vi "3D Primitive Data.vi"(10 "Normal Binding Mode":T1(ring), 11 "Primitive Mode":T3(ring)) -> (1 "Normal Array":cluster{"X":sgl, "Y":sgl, "Z":sgl}[](array[cluster]), 2 "Indices":u32[](array[numeric]), 3 "Vertex Array":cluster{"X":sgl, "Y":sgl, "Z":sgl}[](array[cluster]), 4 "Texture Array":cluster{"X":sgl, "Y":sgl}[](array[cluster]), 5 "Color Array":T2(array[cluster]))   [LabVIEW 2023]
doc: "Create meshes of points for the Using Meshes.vi example. Define some known parameters so the mesh can be processed."
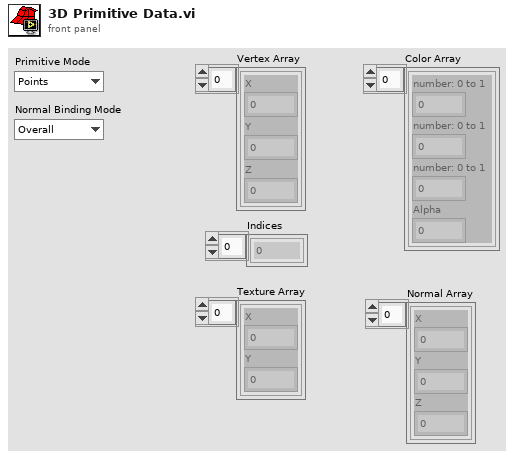
[diagram p1: front panel]
types:
  T1 = enum16{"Overall", "Per Primitive", "Per Vertex", "Binding Off"}
  T2 = cluster{"number: 0 to 1":dbl, "number: 0 to 1":dbl, "number: 0 to 1":dbl, "Alpha":dbl}[]
  T3 = enum16{"Points", "Lines", "Line Strip", "Line Loop", "Triangles", "Triangle Strip", "Triangle Fan", "Quads", "Quad Strip", "Polygon"}
  T4 = cluster{"number: 0 to 1":dbl, "number: 0 to 1":dbl, "number: 0 to 1":dbl}
  T5 = cluster{"number: 0 to 1":dbl, "number: 0 to 1":dbl, "number: 0 to 1":dbl, dbl}
  T6 = cluster{"number: 0 to 1":dbl, "number: 0 to 1":dbl, "number: 0 to 1":dbl, dbl}[]
  T7 = cluster{"number: 0 to 1":dbl, "number: 0 to 1":dbl, "number: 0 to 1":dbl}[]
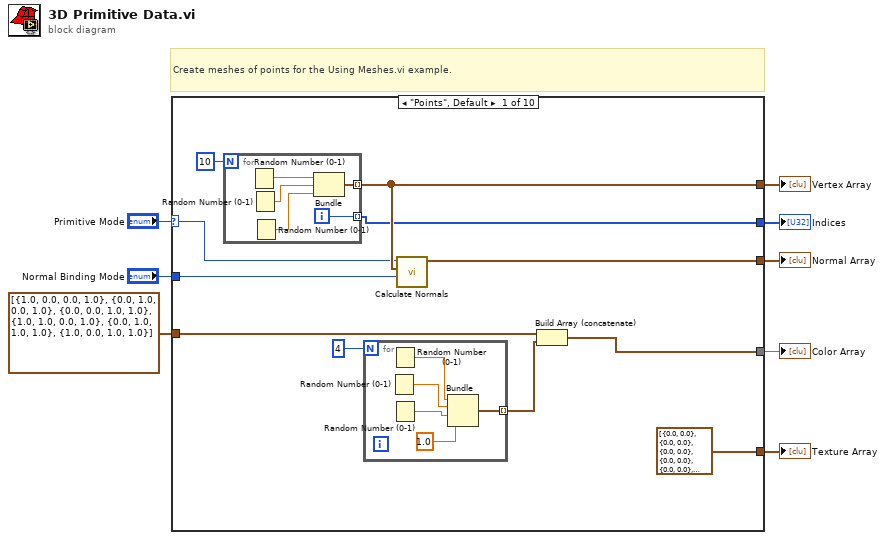
[diagram p0: block diagram]
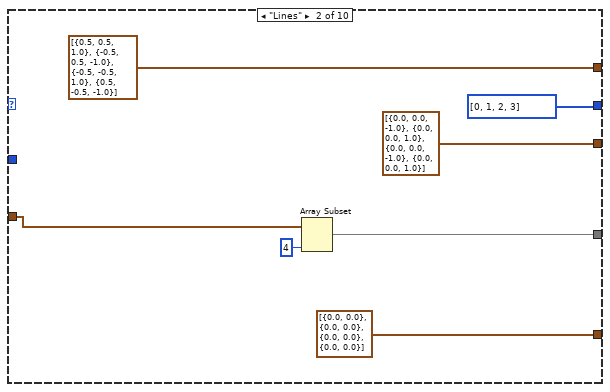
[diagram p2: hidden frame]
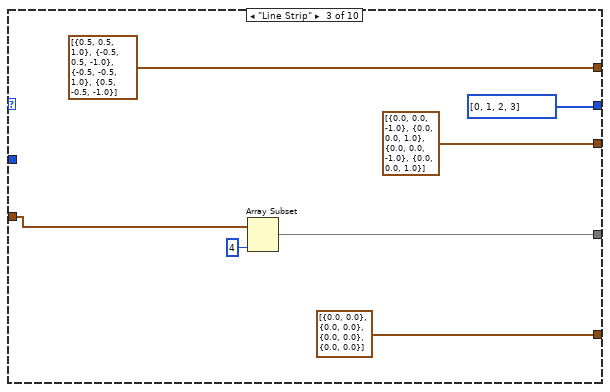
[diagram p3: hidden frame]
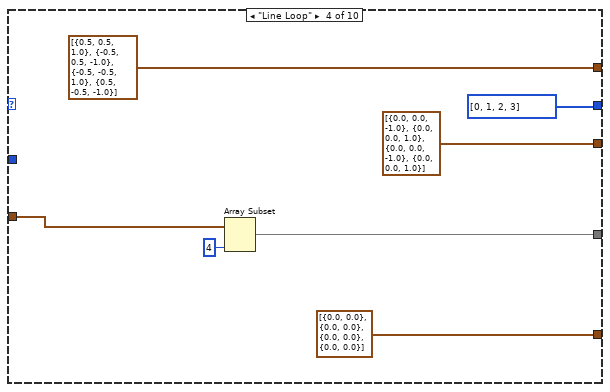
[diagram p4: hidden frame]
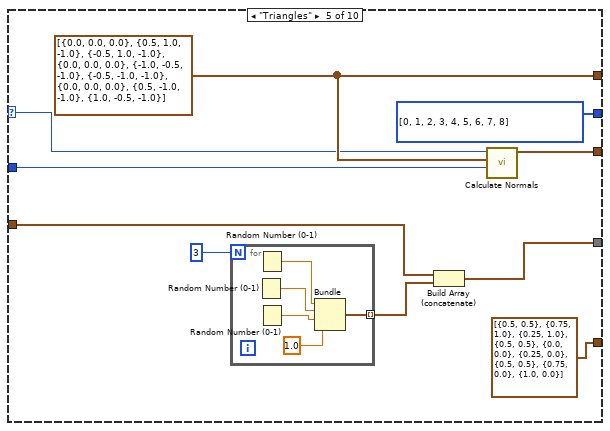
[diagram p5: hidden frame]
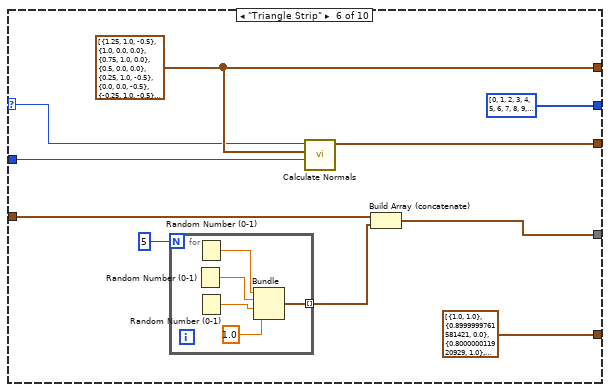
[diagram p6: hidden frame]
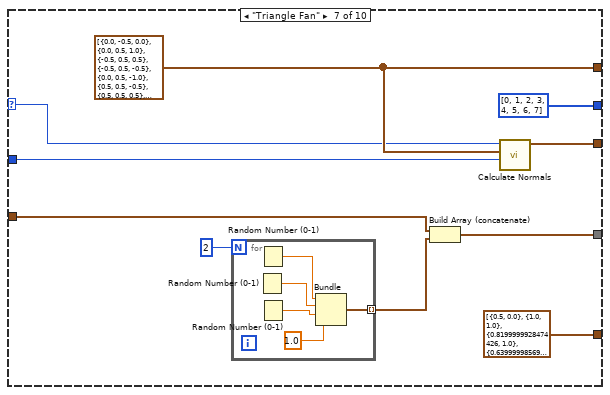
[diagram p7: hidden frame]
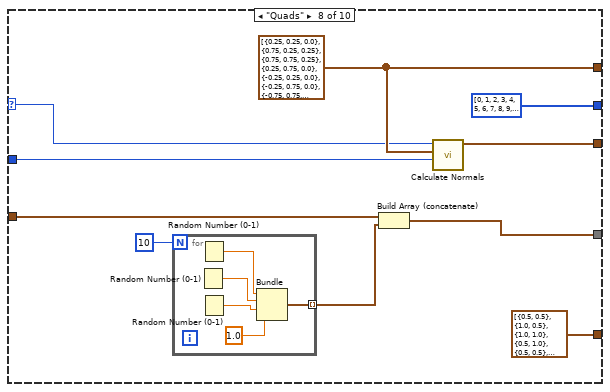
[diagram p8: hidden frame]
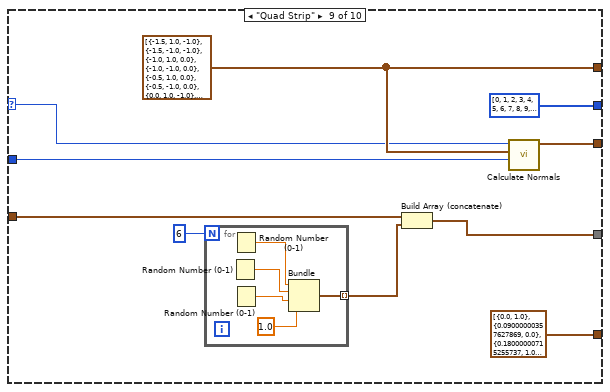
[diagram p9: hidden frame]
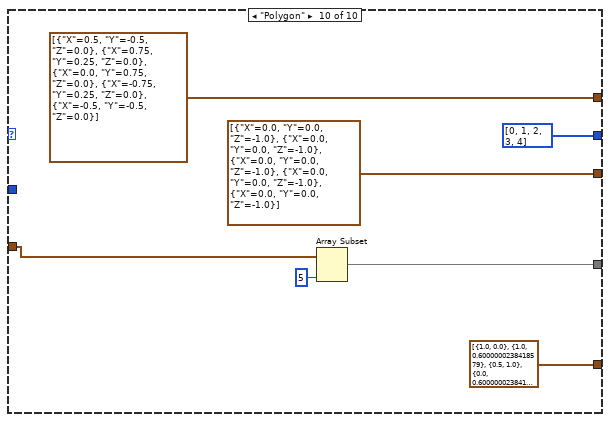
[diagram p10: hidden frame]
diagram:
  # "Create meshes of points for the Using Meshes.vi example."
  n1 = case shown="\"Points\", Default" "Primitive Mode" {
    selector: "Primitive Mode" -> [w9 _ _ _ w51 w66 w81 w96 w111 _]
    tunnel: [w19 cluster{"X":sgl, "Y":sgl, "Z":sgl}[] [{"X"=0.0, "Y"=0.0, "Z"=-1.0}, {"X"=0.0, "Y"=0.0, "Z"=1.0}, {"X"=0.0, "Y"=0.0, "Z"=-1.0}, {"X"=0.0, "Y"=0.0, "Z"=1.0}] cluster{"X":sgl, "Y":sgl, "Z":sgl}[] [{"X"=0.0, "Y"=0.0, "Z"=-1.0}, {"X"=0.0, "Y"=0.0, "Z"=1.0}, {"X"=0.0, "Y"=0.0, "Z"=-1.0}, {"X"=0.0, "Y"=0.0, "Z"=1.0}] cluster{"X":sgl, "Y":sgl, "Z":sgl}[] [{"X"=0.0, "Y"=0.0, "Z"=-1.0}, {"X"=0.0, "Y"=0.0, "Z"=1.0}, {"X"=0.0, "Y"=0.0, "Z"=-1.0}, {"X"=0.0, "Y"=0.0, "Z"=1.0}] w58 w73 w88 w103 w117 cluster{"X":sgl, "Y":sgl, "Z":sgl}[] [{"X"=0.0, "Y"=0.0, "Z"=-1.0}, {"X"=0.0, "Y"=0.0, "Z"=-1.0}, {"X"=0.0, "Y"=0.0, "Z"=-1.0}, {"X"=0.0, "Y"=0.0, "Z"=-1.0}, {"X"=0.0, "Y"=0.0, "Z"=-1.0}]] -> w8
    tunnel: [w17 cluster{"X":sgl, "Y":sgl, "Z":sgl}[] [{"X"=0.5, "Y"=0.5, "Z"=1.0}, {"X"=-0.5, "Y"=0.5, "Z"=-1.0}, {"X"=-0.5, "Y"=-0.5, "Z"=1.0}, {"X"=0.5, "Y"=-0.5, "Z"=-1.0}] ("Vertex Array") cluster{"X":sgl, "Y":sgl, "Z":sgl}[] [{"X"=0.5, "Y"=0.5, "Z"=1.0}, {"X"=-0.5, "Y"=0.5, "Z"=-1.0}, {"X"=-0.5, "Y"=-0.5, "Z"=1.0}, {"X"=0.5, "Y"=-0.5, "Z"=-1.0}] ("Vertex Array") cluster{"X":sgl, "Y":sgl, "Z":sgl}[] [{"X"=0.5, "Y"=0.5, "Z"=1.0}, {"X"=-0.5, "Y"=0.5, "Z"=-1.0}, {"X"=-0.5, "Y"=-0.5, "Z"=1.0}, {"X"=0.5, "Y"=-0.5, "Z"=-1.0}] ("Vertex Array") w57 w74 w87 w102 w118 cluster{"X":sgl, "Y":sgl, "Z":sgl}[] [{"X"=0.5, "Y"=-0.5, "Z"=0.0}, {"X"=0.75, "Y"=0.25, "Z"=0.0}, {"X"=0.0, "Y"=0.75, "Z"=0.0}, {"X"=-0.75, "Y"=0.25, "Z"=0.0}, {"X"=-0.5, "Y"=-0.5, "Z"=0.0}] ("Vertex Array")] -> w6
    tunnel: [w10 w30 w37 w44 w54 w67 w83 w97 w112 w126] -> w5
    tunnel: [cluster{"X":sgl, "Y":sgl}[] [{"X"=0.0, "Y"=0.0}, {"X"=0.0, "Y"=0.0}, {"X"=0.0, "Y"=0.0}, {"X"=0.0, "Y"=0.0}, {"X"=0.0, "Y"=0.0}, {"X"=0.0, "Y"=0.0}, {"X"=0.0, "Y"=0.0}, {"X"=0.0, "Y"=0.0}, {"X"=0.0, "Y"=0.0}, {"X"=0.0, "Y"=0.0}] ("Texture Array") cluster{"X":sgl, "Y":sgl}[] [{"X"=0.0, "Y"=0.0}, {"X"=0.0, "Y"=0.0}, {"X"=0.0, "Y"=0.0}, {"X"=0.0, "Y"=0.0}] ("Vertex Array") cluster{"X":sgl, "Y":sgl}[] [{"X"=0.0, "Y"=0.0}, {"X"=0.0, "Y"=0.0}, {"X"=0.0, "Y"=0.0}, {"X"=0.0, "Y"=0.0}] ("Vertex Array") cluster{"X":sgl, "Y":sgl}[] [{"X"=0.0, "Y"=0.0}, {"X"=0.0, "Y"=0.0}, {"X"=0.0, "Y"=0.0}, {"X"=0.0, "Y"=0.0}] ("Vertex Array") cluster{"X":sgl, "Y":sgl}[] [{"X"=0.5, "Y"=0.5}, {"X"=0.75, "Y"=1.0}, {"X"=0.25, "Y"=1.0}, {"X"=0.5, "Y"=0.5}, {"X"=0.0, "Y"=0.0}, {"X"=0.25, "Y"=0.0}, {"X"=0.5, "Y"=0.5}, {"X"=0.75, "Y"=0.0}, {"X"=1.0, "Y"=0.0}] ("Vertex Array") cluster{"X":sgl, "Y":sgl}[] [{"X"=1.0, "Y"=1.0}, {"X"=0.9, "Y"=0.0}, {"X"=0.8, "Y"=1.0}, {"X"=0.7, "Y"=0.0}, {"X"=0.6, "Y"=1.0}, {"X"=0.5, "Y"=0.0}, {"X"=0.4, "Y"=1.0}, {"X"=0.3, "Y"=0.0}, {"X"=0.2, "Y"=1.0}, {"X"=0.1, "Y"=0.0}, {"X"=0.0, "Y"=1.0}] ("Vertex Array") cluster{"X":sgl, "Y":sgl}[] [{"X"=0.5, "Y"=0.0}, {"X"=1.0, "Y"=1.0}, {"X"=0.82, "Y"=1.0}, {"X"=0.64, "Y"=1.0}, {"X"=0.48, "Y"=1.0}, {"X"=0.32, "Y"=1.0}, {"X"=0.16, "Y"=1.0}, {"X"=1.0, "Y"=1.0}] ("Vertex Array") cluster{"X":sgl, "Y":sgl}[] [{"X"=0.5, "Y"=0.5}, {"X"=1.0, "Y"=0.5}, {"X"=1.0, "Y"=1.0}, {"X"=0.5, "Y"=1.0}, {"X"=0.5, "Y"=0.5}, {"X"=0.5, "Y"=1.0}, {"X"=0.0, "Y"=1.0}, {"X"=0.0, "Y"=0.5}, {"X"=0.5, "Y"=0.5}, {"X"=0.0, "Y"=0.5}, {"X"=0.0, "Y"=0.0}, {"X"=0.5, "Y"=0.0}, {"X"=0.5, "Y"=0.5}, {"X"=0.5, "Y"=0.0}, {"X"=1.0, "Y"=0.0}, {"X"=1.0, "Y"=0.5}] ("Vertex Array") cluster{"X":sgl, "Y":sgl}[] [{"X"=0.0, "Y"=1.0}, {"X"=0.09, "Y"=0.0}, {"X"=0.18, "Y"=1.0}, {"X"=0.27, "Y"=0.0}, {"X"=0.36, "Y"=1.0}, {"X"=0.45, "Y"=0.0}, {"X"=0.54, "Y"=1.0}, {"X"=0.63, "Y"=0.0}, {"X"=0.72, "Y"=1.0}, {"X"=0.81, "Y"=0.0}, {"X"=0.9, "Y"=1.0}, {"X"=1.0, "Y"=0.0}] ("Vertex Array") cluster{"X":sgl, "Y":sgl}[] [{"X"=1.0, "Y"=0.0}, {"X"=1.0, "Y"=0.6}, {"X"=0.5, "Y"=1.0}, {"X"=0.0, "Y"=0.6}, {"X"=0.0, "Y"=0.0}] ("Vertex Array")] -> w4
    tunnel: [w15 u32[] [0, 1, 2, 3] ("Indices") u32[] [0, 1, 2, 3] ("Indices") u32[] [0, 1, 2, 3] ("Indices") u32[] [0, 1, 2, 3, 4, 5, 6, 7, 8] ("Indices") u32[] [0, 1, 2, 3, 4, 5, 6, 7, 8, 9, 10] ("Indices") u32[] [0, 1, 2, 3, 4, 5, 6, 7] ("Indices") u32[] [0, 1, 2, 3, 4, 5, 6, 7, 8, 9, 10, 11, 12, 13, 14, 15] ("Indices") u32[] [0, 1, 2, 3, 4, 5, 6, 7, 8, 9, 10, 11] ("Indices") u32[] [0, 1, 2, 3, 4] ("Indices")] -> w3
    tunnel: "Normal Binding Mode" -> [w14 _ _ _ w55 w71 w86 w101 w116 _]
    tunnel: cluster{dbl, dbl, dbl, dbl}[] [{1.0, 0.0, 0.0, 1.0}, {0.0, 1.0, 0.0, 1.0}, {0.0, 0.0, 1.0, 1.0}, {1.0, 1.0, 0.0, 1.0}, {0.0, 1.0, 1.0, 1.0}, {1.0, 0.0, 1.0, 1.0}] -> [w13 w32 w39 w46 w53 w69 w84 w99 w114 w128]
    frame "Points", Default {
      n2 = for {
        N: 10 -> [_]
        tunnel: [w27] -> w17 mode=indexing
        tunnel: [w26] -> w15 mode=indexing
        i -> [w26]
        n3 = Random Number (0-1)() -> (number: 0 to 1=w29:dbl)
        n4 = Random Number (0-1)() -> (number: 0 to 1=w28:dbl)
        n5 = Random Number (0-1)() -> (number: 0 to 1=w25:dbl)
        n6 = Bundle("number: 0 to 1"=w29, "number: 0 to 1"=w28, "number: 0 to 1"=w25) -> (w27:T4)  [unwired: 1 in]
      }
      n7 = for {
        N: 4 -> [_]
        tunnel: [w24] -> w11 mode=indexing
        n8 = Random Number (0-1)() -> (number: 0 to 1=w21:dbl)
        n9 = Random Number (0-1)() -> (number: 0 to 1=w22:dbl)
        n10 = Random Number (0-1)() -> (number: 0 to 1=w20:dbl)
        n11 = Bundle("number: 0 to 1"=w22, "number: 0 to 1"=w21, "number: 0 to 1"=w20, 1.0) -> (w24:T5)  [unwired: 1 in]
      }
      n12 = call "Calculate Normals.vi"("Color Binding Mode"=w14, "Vertex Array"=w17, "Draw Mode"=w9) -> ("Normal Array"=w19:cluster{"X":sgl, "Y":sgl, "Z":sgl}[])  [unwired: 8 in]
      n13 = Build Array (concatenate)(w13, w11) -> (w10:T6)
    }
    frame "Lines" {
      n14 = Array Subset(array=w32, length=4) -> (w30:cluster{dbl, dbl, dbl, dbl}[])  [unwired: 1 in]
    }
    frame "Line Strip" {
      n15 = Array Subset(array=w39, length=4) -> (w37:cluster{dbl, dbl, dbl, dbl}[])  [unwired: 1 in]
    }
    frame "Line Loop" {
      n16 = Array Subset(array=w46, length=4) -> (w44:cluster{dbl, dbl, dbl, dbl}[])  [unwired: 1 in]
    }
    frame "Triangles" {
      w57 = cluster{"X":sgl, "Y":sgl, "Z":sgl}[] [{"X"=0.0, "Y"=0.0, "Z"=0.0}, {"X"=0.5, "Y"=1.0, "Z"=-1.0}, {"X"=-0.5, "Y"=1.0, "Z"=-1.0}, {"X"=0.0, "Y"=0.0, "Z"=0.0}, {"X"=-1.0, "Y"=-0.5, "Z"=-1.0}, {"X"=-0.5, "Y"=-1.0, "Z"=-1.0}, {"X"=0.0, "Y"=0.0, "Z"=0.0}, {"X"=0.5, "Y"=-1.0, "Z"=-1.0}, {"X"=1.0, "Y"=-0.5, "Z"=-1.0}] ("Vertex Array")
      n17 = for {
        N: 3 -> [_]
        tunnel: [w65] -> w52 mode=indexing
        n18 = Random Number (0-1)() -> (number: 0 to 1=w62:dbl)
        n19 = Random Number (0-1)() -> (number: 0 to 1=w63:dbl)
        n20 = Random Number (0-1)() -> (number: 0 to 1=w61:dbl)
        n21 = Bundle("number: 0 to 1"=w63, "number: 0 to 1"=w62, "number: 0 to 1"=w61, 1.0) -> (w65:T5)  [unwired: 1 in]
      }
      n22 = Build Array (concatenate)(w53, w52) -> (w54:T6)
      n23 = call "Calculate Normals.vi"("Color Binding Mode"=w55, "Vertex Array"=w57, "Draw Mode"=w51) -> ("Normal Array"=w58:cluster{"X":sgl, "Y":sgl, "Z":sgl}[])  [unwired: 8 in]
    }
    frame "Triangle Strip" {
      w74 = cluster{"X":sgl, "Y":sgl, "Z":sgl}[] [{"X"=1.25, "Y"=1.0, "Z"=-0.5}, {"X"=1.0, "Y"=0.0, "Z"=0.0}, {"X"=0.75, "Y"=1.0, "Z"=0.0}, {"X"=0.5, "Y"=0.0, "Z"=0.0}, {"X"=0.25, "Y"=1.0, "Z"=-0.5}, {"X"=0.0, "Y"=0.0, "Z"=-0.5}, {"X"=-0.25, "Y"=1.0, "Z"=-0.5}, {"X"=-0.5, "Y"=0.0, "Z"=0.0}, {"X"=-0.75, "Y"=1.0, "Z"=0.0}, {"X"=-1.0, "Y"=0.0, "Z"=0.0}, {"X"=-1.25, "Y"=1.0, "Z"=-0.5}] ("Vertex Array")
      n24 = for {
        N: 5 -> [_]
        tunnel: [w80] -> w68 mode=indexing
        n25 = Random Number (0-1)() -> (number: 0 to 1=w77:dbl)
        n26 = Random Number (0-1)() -> (number: 0 to 1=w78:dbl)
        n27 = Random Number (0-1)() -> (number: 0 to 1=w76:dbl)
        n28 = Bundle("number: 0 to 1"=w78, "number: 0 to 1"=w77, "number: 0 to 1"=w76, 1.0) -> (w80:T5)  [unwired: 1 in]
      }
      n29 = call "Calculate Normals.vi"("Color Binding Mode"=w71, "Vertex Array"=w74, "Draw Mode"=w66) -> ("Normal Array"=w73:cluster{"X":sgl, "Y":sgl, "Z":sgl}[])  [unwired: 8 in]
      n30 = Build Array (concatenate)(w69, w68) -> (w67:T6)
    }
    frame "Triangle Fan" {
      w87 = cluster{"X":sgl, "Y":sgl, dbl}[] [{"X"=0.0, "Y"=-0.5, 0.0}, {"X"=0.0, "Y"=0.5, 1.0}, {"X"=-0.5, "Y"=0.5, 0.5}, {"X"=-0.5, "Y"=0.5, -0.5}, {"X"=0.0, "Y"=0.5, -1.0}, {"X"=0.5, "Y"=0.5, -0.5}, {"X"=0.5, "Y"=0.5, 0.5}, {"X"=0.0, "Y"=0.5, 1.0}] ("Vertex Array")
      n31 = for {
        N: 2 -> [_]
        tunnel: [w95] -> w82 mode=indexing
        n32 = Random Number (0-1)() -> (number: 0 to 1=w92:dbl)
        n33 = Random Number (0-1)() -> (number: 0 to 1=w93:dbl)
        n34 = Random Number (0-1)() -> (number: 0 to 1=w91:dbl)
        n35 = Bundle("number: 0 to 1"=w93, "number: 0 to 1"=w92, "number: 0 to 1"=w91, 1.0) -> (w95:T5)  [unwired: 1 in]
      }
      n36 = Build Array (concatenate)(w84, w82) -> (w83:T6)
      n37 = call "Calculate Normals.vi"("Color Binding Mode"=w86, "Vertex Array"=w87, "Draw Mode"=w81) -> ("Normal Array"=w88:cluster{"X":sgl, "Y":sgl, "Z":sgl}[])  [unwired: 8 in]
    }
    frame "Quads" {
      w102 = T7 [{"number: 0 to 1"=0.25, "number: 0 to 1"=0.25, "number: 0 to 1"=0.0}, {"number: 0 to 1"=0.75, "number: 0 to 1"=0.25, "number: 0 to 1"=0.25}, {"number: 0 to 1"=0.75, "number: 0 to 1"=0.75, "number: 0 to 1"=0.25}, {"number: 0 to 1"=0.25, "number: 0 to 1"=0.75, "number: 0 to 1"=0.0}, {"number: 0 to 1"=-0.25, "number: 0 to 1"=0.25, "number: 0 to 1"=0.0}, {"number: 0 to 1"=-0.25, "number: 0 to 1"=0.75, "number: 0 to 1"=0.0}, {"number: 0 to 1"=-0.75, "number: 0 to 1"=0.75, "number: 0 to 1"=0.25}, {"number: 0 to 1"=-0.75, "number: 0 to 1"=0.25, "number: 0 to 1"=0.25}, {"number: 0 to 1"=-0.25, "number: 0 to 1"=-0.25, "number: 0 to 1"=0.0}, {"number: 0 to 1"=-0.75, "number: 0 to 1"=-0.25, "number: 0 to 1"=0.25}, {"number: 0 to 1"=-0.75, "number: 0 to 1"=-0.75, "number: 0 to 1"=0.25}, {"number: 0 to 1"=-0.25, "number: 0 to 1"=-0.75, "number: 0 to 1"=0.0}, {"number: 0 to 1"=0.25, "number: 0 to 1"=-0.25, "number: 0 to 1"=0.0}, {"number: 0 to 1"=0.25, "number: 0 to 1"=-0.75, "number: 0 to 1"=0.0}, {"number: 0 to 1"=0.75, "number: 0 to 1"=-0.75, "number: 0 to 1"=0.25}, {"number: 0 to 1"=0.75, "number: 0 to 1"=-0.25, "number: 0 to 1"=0.25}] ("Vertex Array")
      n38 = for {
        N: 10 -> [_]
        tunnel: [w110] -> w98 mode=indexing
        n39 = Random Number (0-1)() -> (number: 0 to 1=w107:dbl)
        n40 = Random Number (0-1)() -> (number: 0 to 1=w108:dbl)
        n41 = Random Number (0-1)() -> (number: 0 to 1=w106:dbl)
        n42 = Bundle("number: 0 to 1"=w108, "number: 0 to 1"=w107, "number: 0 to 1"=w106, 1.0) -> (w110:T5)  [unwired: 1 in]
      }
      n43 = Build Array (concatenate)(w99, w98) -> (w97:T6)
      n44 = call "Calculate Normals.vi"("Color Binding Mode"=w101, "Vertex Array"=w102, "Draw Mode"=w96) -> ("Normal Array"=w103:cluster{"X":sgl, "Y":sgl, "Z":sgl}[])  [unwired: 8 in]
    }
    frame "Quad Strip" {
      w118 = cluster{"X":sgl, "Y":sgl, "Z":sgl}[] [{"X"=-1.5, "Y"=1.0, "Z"=-1.0}, {"X"=-1.5, "Y"=-1.0, "Z"=-1.0}, {"X"=-1.0, "Y"=1.0, "Z"=0.0}, {"X"=-1.0, "Y"=-1.0, "Z"=0.0}, {"X"=-0.5, "Y"=1.0, "Z"=0.0}, {"X"=-0.5, "Y"=-1.0, "Z"=0.0}, {"X"=0.0, "Y"=1.0, "Z"=-1.0}, {"X"=0.0, "Y"=-1.0, "Z"=-1.0}, {"X"=0.5, "Y"=1.0, "Z"=-1.0}, {"X"=0.5, "Y"=-1.0, "Z"=-1.0}, {"X"=1.0, "Y"=1.0, "Z"=-1.0}, {"X"=1.0, "Y"=-1.0, "Z"=-1.0}] ("Vertex Array")
      n45 = for {
        N: 6 -> [_]
        tunnel: [w125] -> w113 mode=indexing
        n46 = Random Number (0-1)() -> (number: 0 to 1=w122:dbl)
        n47 = Random Number (0-1)() -> (number: 0 to 1=w123:dbl)
        n48 = Random Number (0-1)() -> (number: 0 to 1=w121:dbl)
        n49 = Bundle("number: 0 to 1"=w123, "number: 0 to 1"=w122, "number: 0 to 1"=w121, 1.0) -> (w125:T5)  [unwired: 1 in]
      }
      n50 = Build Array (concatenate)(w114, w113) -> (w112:T6)
      n51 = call "Calculate Normals.vi"("Color Binding Mode"=w116, "Vertex Array"=w118, "Draw Mode"=w111) -> ("Normal Array"=w117:cluster{"X":sgl, "Y":sgl, "Z":sgl}[])  [unwired: 8 in]
    }
    frame "Polygon" {
      n52 = Array Subset(array=w128, length=5) -> (w126:cluster{dbl, dbl, dbl, dbl}[])  [unwired: 1 in]
    }
  }
  "Vertex Array" <- w6
  "Color Array" <- w5
  "Texture Array" <- w4
  "Normal Array" <- w8
  "Indices" <- w3
